vi "条形码扫描窗口.vi"(1 "扫描的ID号":string) -> (0 "ID显示":string)   [LabVIEW 2014]
panel:
  in  "确定":bool
  # "该产品ID如下"
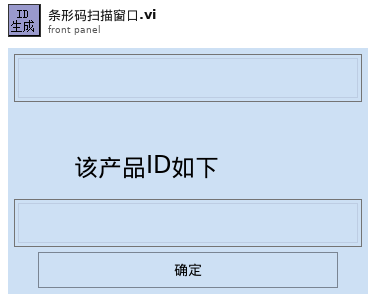
[diagram p1: front panel]
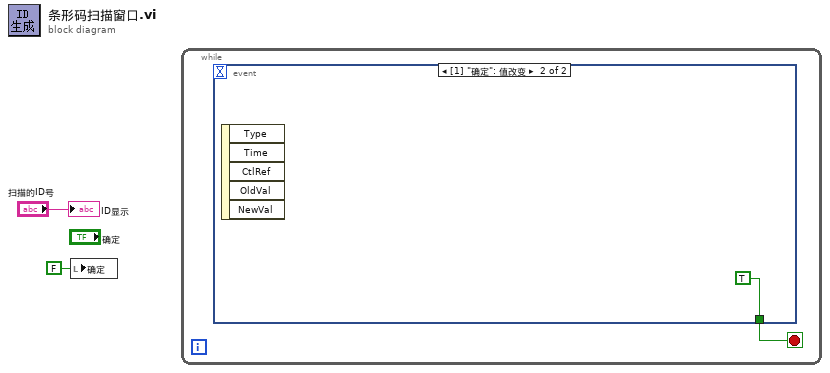
[diagram p0: block diagram]
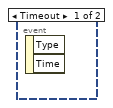
[diagram p2: hidden frame]
diagram:
  n1 = local write "确定"(FALSE ("确定")) -> ()
  n2 = while {
    stop <- w3 stop-if-true
    n3 = event shown="[1] \"确定\": 值改变" {
      selector: _ -> [_ _]
      dyn-events: _ -> [_ _]
      timeout: _ -> [_ _]
      tunnel: [_ TRUE] -> w3
      event Timeout {
        n4 = event-data() -> ()  [unwired: 1 in, 2 out]
      }
      event "确定": Value Change {
        n5 = event-data() -> ()  [unwired: 1 in, 5 out]
      }
    }
  }
  "ID显示" <- "扫描的ID号"
